vi "RESET.vi"(1 "SPI Config In":T1) -> (0 "SPI Config Out":T1)   [LabVIEW 2019]
uses:
  SPI/SPI Config.ctl
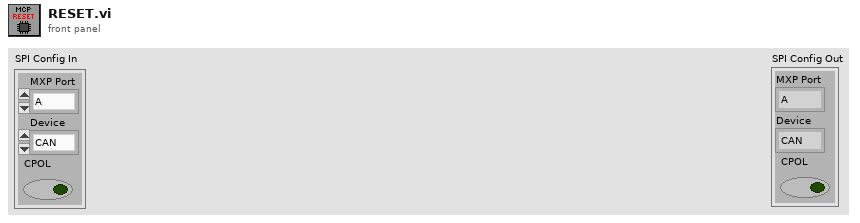
[diagram p1: front panel]
types:
  T1 = typedef "SPI Config.ctl" = cluster{"MXP Port":enum16{"A", "B"}, "Device":enum16{"CAN", "ENC", "IMU1", "IMU2"}, "CPOL":bool}
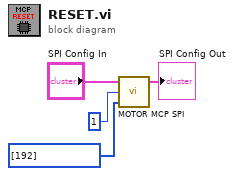
[diagram p0: block diagram]
diagram:
  n1 = call "MOTOR MCP SPI.vi"("Data to Write"=u8[] [192], "Frames to Write"=u8 1, "SPI Config In"="SPI Config In") -> ("SPI Config Out"=→"SPI Config Out":T1)  [unwired: 2 out]
